vi "Oszilloscope_Bildschirmanpassung.vi"() -> ()   [LabVIEW 2016]
panel:
  out "Lesepuffer 3":string
  out "Lesepuffer 2":string
  out "VISA resource name out":refnum<visa-resource-name>
  in  "VISA-Ressourcenname":refnum<visa-resource-name>
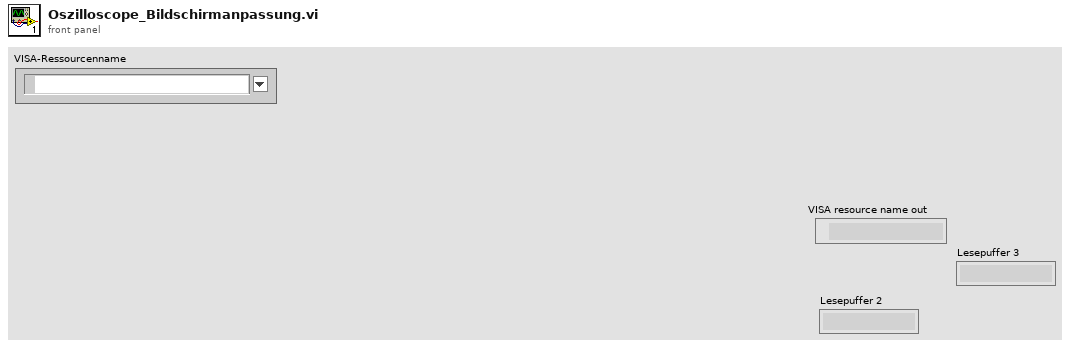
[diagram p1: front panel]
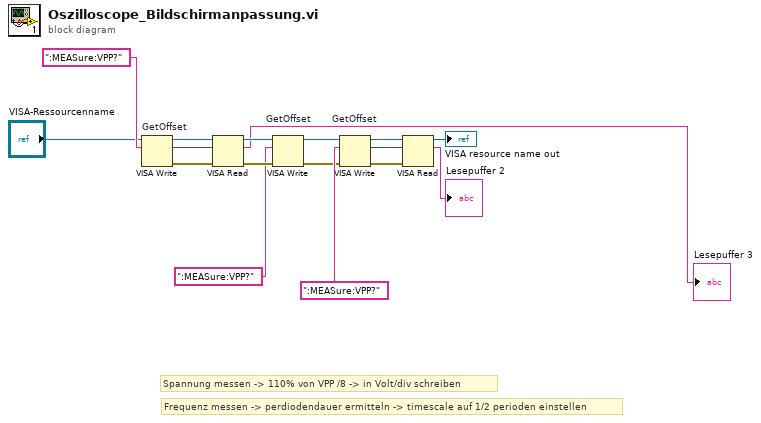
[diagram p0: block diagram]
diagram:
  # "Frequenz messen -> perdiodendauer ermitteln -> timescale auf 1/2 perioden einstellen"
  # "Spannung messen -> 110% von VPP /8 -> in Volt/div schreiben"
  n1 = VISA Write "GetOffset"(VISA resource name="VISA-Ressourcenname", write buffer=":MEASure:VPP?" ("Schreibpuffer")) -> (VISA resource name out=w17:refnum<visa-resource-name>, return count=w14:u32, error out=w16:errorcluster)  [unwired: 1 in]
  n2 = VISA Read(VISA resource name=w17, byte count=w14, error in (no error)=w16) -> (VISA resource name out=w6:refnum<visa-resource-name>, read buffer=→"Lesepuffer 3":string, error out=w5:errorcluster)  [unwired: 1 out]
  n3 = VISA Write "GetOffset"(VISA resource name=w6, write buffer=":MEASure:VPP?" ("Schreibpuffer"), error in (no error)=w5) -> (VISA resource name out=w4:refnum<visa-resource-name>, error out=w3:errorcluster)  [unwired: 1 out]
  n4 = VISA Write "GetOffset"(VISA resource name=w4, write buffer=":MEASure:VPP?" ("Schreibpuffer"), error in (no error)=w3) -> (VISA resource name out=w8:refnum<visa-resource-name>, return count=w11:u32, error out=w9:errorcluster)
  n5 = VISA Read(VISA resource name=w8, byte count=w11, error in (no error)=w9) -> (VISA resource name out=→"VISA resource name out":refnum<visa-resource-name>, read buffer=→"Lesepuffer 2":string)  [unwired: 2 out]
